vi "svx_SpecifiedMaxMinDecimateDBL1DArray.vi"(10 "decimation factor":i32, 11 "DBL Array":dbl[](array[numeric]) format="%.2f") -> (1 "actual decimation":dbl format="%.2f", 2 "decimated array":dbl[](array[numeric]) format="%.2f", 3 "dup DBL Array":dbl[](array[numeric]) format="%.2f")   [LabVIEW 2017, in "SVX Waterfall Graph.xctl"]
doc: "Decimate an array before it is sent to the graph object so that processing time and memory are saved."
uses:
  <vilib>/addons/_XControls/Waterfall Graph/SVX Waterfall Graph.xctl
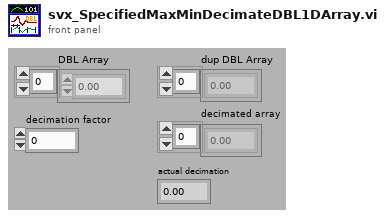
[diagram p1: front panel]
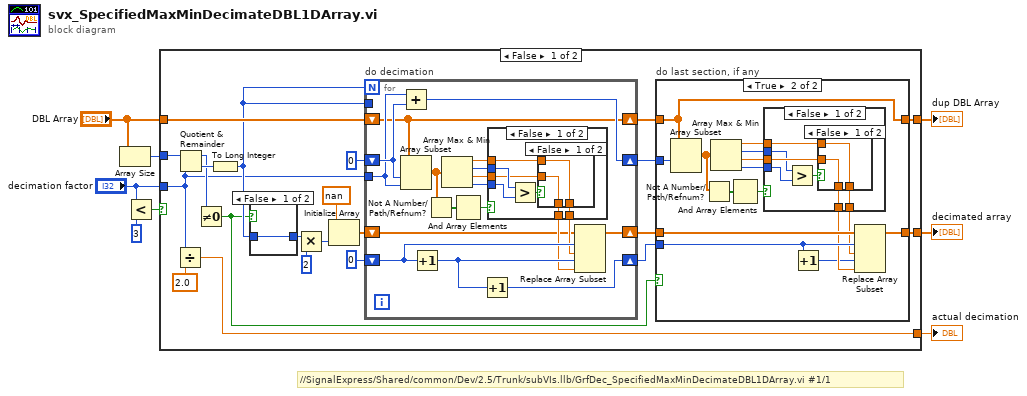
[diagram p0: block diagram]
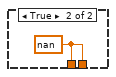
[diagram p4: hidden frame]
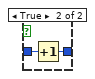
[diagram p5: hidden frame]
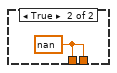
[diagram p7: hidden frame]
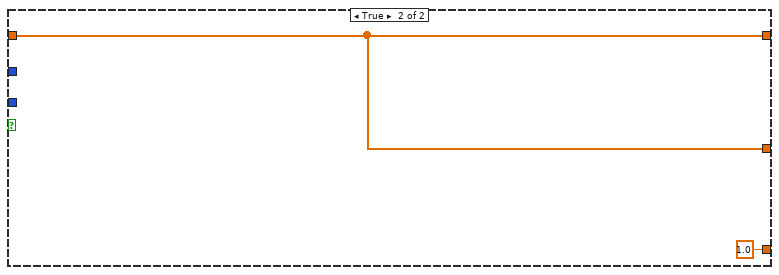
[diagram p8: hidden frame]
diagram:
  # "//SignalExpress/Shared/common/Dev/2.5/Trunk/subVIs.llb/GrfDec_SpecifiedMaxMinDecimateDBL1DArray.vi #1/1"
  n1 = Array Size(array="DBL Array") -> (size(s)=w6:i32)
  n2 = Less?(x="decimation factor", y=3) -> (x < y?=w1:bool)
  n3 = case shown="False" w1 {
    tunnel: "DBL Array" -> [w30 w94]
    tunnel: [w29 w94] -> w7
    tunnel: w6 -> [w28 _]
    tunnel: [w27 1.0] -> w5
    tunnel: "decimation factor" -> [w10 _]
    tunnel: [w9 w94] -> w2
    frame False {
      n4 = Divide(x=w10, y=2.0) -> (x/y=w27:dbl)
      n5 = Quotient & Remainder(x=w28, y=w10) -> (x-y*floor(x/y)=w16:i32, floor(x/y)=w17:i32)
      n6 = Not Equal To 0?(x=w16) -> (x != 0?=w13:bool)
      n7 = To Long Integer(number=w17) -> (32bit integer=w14:i32)
      n8 = case shown="False" w13 {
        tunnel: [w60 w62] -> w15
        tunnel: w14 -> [w60 w61]
        frame False {
        }
        frame True {
          n9 = Increment(x=w61) -> (x+1=w62:i32)
        }
      }
      n10 = Multiply(x=w15, y=2) -> (x*y=w22:i32)
      n11 = Initialize Array(nan, w22) -> (w21:dbl[])
      n12 = for "do decimation" {
        N: w14 -> [_]
        shift-right: [w79] -> w18
        shift-left: 0 ("32bit integer") -> [w80]
        shift-right: [w67] -> w20
        shift-left: 0 ("32bit integer") -> [w77]
        tunnel: w14 -> [_]
        tunnel: w10 -> [w70]
        shift-right: [w68] -> w19
        shift-left: w21 -> [w69]
        shift-right: [w66] -> w11
        shift-left: w30 -> [w66]
        n13 = Add(x=w70, y=w77) -> (x+y=w67:i32)
        n14 = Array Subset(array=w66, index=w77, length=w70) -> (w65:dbl[])
        n15 = Increment(x=w80) -> (x+1=w78:i32)
        n16 = Not A Number/Path/Refnum?(number/path/refnum=w65) -> (NaN/Path/Refnum?=w64:bool[])
        n17 = Array Max & Min(array=w65) -> (max value=w73:dbl, max index (indices)=w76:i32, min value=w74:dbl, min index (indices)=w75:i32)
        n18 = And Array Elements(Boolean array=w64) -> (logical AND=w63:bool)
        n19 = Increment(x=w78) -> (x+1=w79:i32)
        n20 = case shown="False" w63 {
          tunnel: w76 -> [w86 _]
          tunnel: w75 -> [w85 _]
          tunnel: w74 -> [w84 _]
          tunnel: w73 -> [w83 _]
          tunnel: [w82 w92] -> w72
          tunnel: [w81 w92] -> w71
          frame False {
            n21 = Greater?(x=w86, y=w85) -> (0:w87:bool)
            n22 = case shown="False" w87 {
              tunnel: w84 -> [w88 w91]
              tunnel: w83 -> [w89 w90]
              tunnel: [w89 w91] -> w82
              tunnel: [w88 w90] -> w81
              frame False {
              }
              frame True {
              }
            }
          }
          frame True {
            w92 = nan
          }
        }
        n23 = Replace Array Subset(array=w69, new element #1=w72, index #1=w80, new element #2=w71, index #2=w78) -> (w68:dbl[])
      }
      n24 = case "do last section, if any" shown="True" w13 {
        tunnel: w20 -> [_ w47]
        tunnel: w11 -> [w31 w33]
        tunnel: w19 -> [w32 w46]
        tunnel: [w32 w37] -> w29
        tunnel: w18 -> [_ w45]
        tunnel: [w31 w33] -> w9
        frame False {
        }
        frame True {
          n25 = Array Subset(array=w33, index=w47) -> (w35:dbl[])  [unwired: 1 in]
          n26 = Not A Number/Path/Refnum?(number/path/refnum=w35) -> (NaN/Path/Refnum?=w36:bool[])
          n27 = Array Max & Min(array=w35) -> (max value=w43:dbl, max index (indices)=w40:i32, min value=w42:dbl, min index (indices)=w41:i32)
          n28 = And Array Elements(Boolean array=w36) -> (logical AND=w34:bool)
          n29 = case shown="False" w34 {
            tunnel: [w54 w59] -> w44
            tunnel: w43 -> [w53 _]
            tunnel: w42 -> [w52 _]
            tunnel: w41 -> [w51 _]
            tunnel: w40 -> [w50 _]
            tunnel: [w48 w59] -> w39
            frame False {
              n30 = Greater?(x=w50, y=w51) -> (0:w49:bool)
              n31 = case shown="False" w49 {
                tunnel: w52 -> [w55 w58]
                tunnel: w53 -> [w56 w57]
                tunnel: [w56 w58] -> w54
                tunnel: [w55 w57] -> w48
                frame False {
                }
                frame True {
                }
              }
            }
            frame True {
              w59 = nan
            }
          }
          n32 = Increment(x=w45) -> (x+1=w38:i32)
          n33 = Replace Array Subset(array=w46, new element #1=w44, index #1=w45, new element #2=w39, index #2=w38) -> (w37:dbl[])
        }
      }
    }
    frame True {
    }
  }
  "decimated array" <- w7
  "actual decimation" <- w5
  "dup DBL Array" <- w2
